vi "Heartbeat Checker.vi"(8 "Error In":errorcluster, 10 "Interval":i32=1000 format="%d ms", 11 "reference in":refnum<class "Network Mangement.lvclass">) -> ()   [LabVIEW 2024, in "Network Mangement.lvclass"]
uses:
  Network Mangement.lvclass
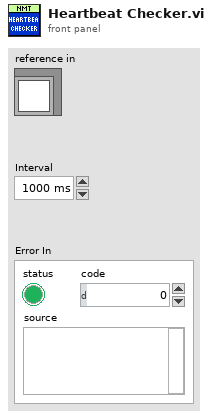
[diagram p1: front panel]
types:
  T1 = cluster{"Timeouted Heartbeat":cluster{"Node-ID":u8, "Heartbeat":cluster{"Period":u16, "Timeout":u16, "Last Beat":timestamp}}}
  T2 = typedef "Network Mangement.lvclass/ObjectAttributes.ctl" = cluster{"Nodes":map{u8, u8}, "Heartbeats":map{u8, cluster{"Period":u16, "Timeout":u16, "Last Beat":timestamp}}, "Events":cluster{"Stop Heartbeat Checker":refnum<user-event>, "Heartbeat Timeout":refnum<user-event>, "Heartbeat Checker Error":refnum<user-event>}, "Heartbeat Checker":refnum<vi>}
  T3 = map{u8, cluster{"Period":u16, "Timeout":u16, "Last Beat":timestamp}}
  T4 = cluster{"Period":u16, "Timeout":u16, "Last Beat":timestamp}
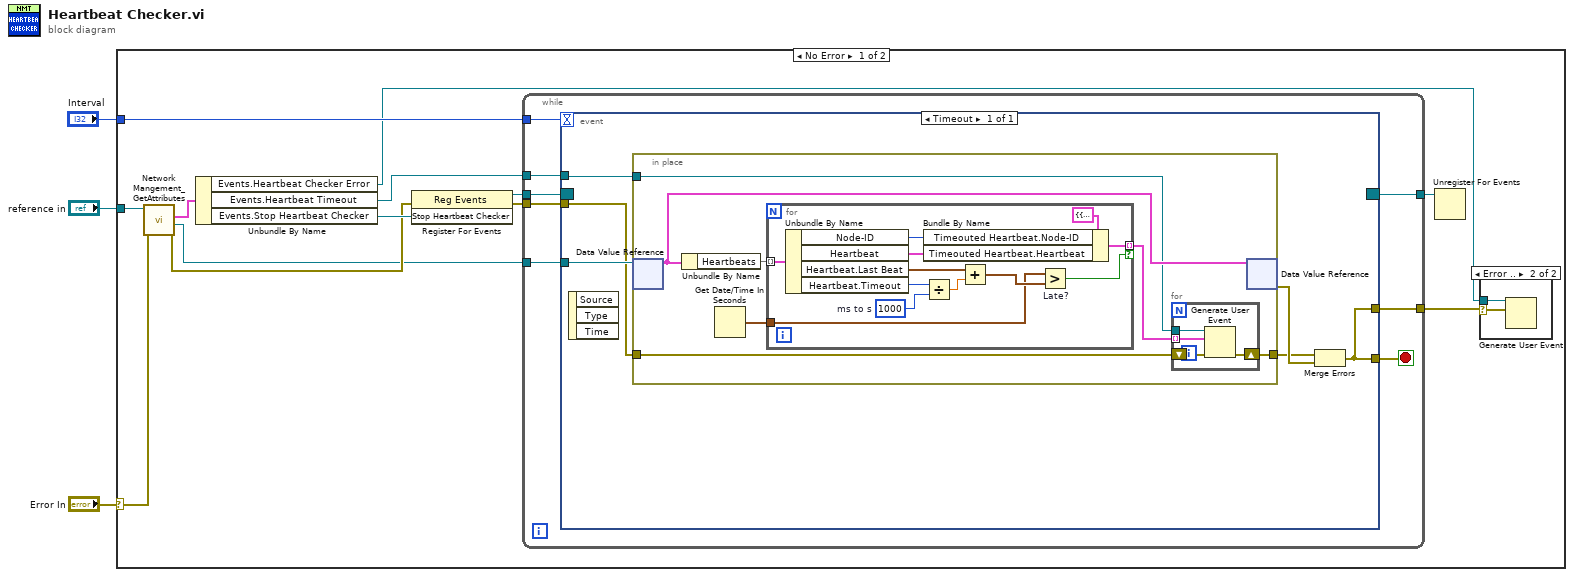
[diagram p0: block diagram]
diagram:
  n1 = case shown="No Error" "Error In" {
    selector: "Error In" -> [w16 _]
    tunnel: "reference in" -> [w14 _]
    tunnel: "Interval" -> [w10 _]
    frame No Error {
      n2 = call "Network Mangement_GetAttributes.vi"("Error In"=w16, "reference in"=w14) -> ("Error Out"=w12:errorcluster, "DataRef"=w8:refnum<data-value>, "Data"=w15:T2)  [unwired: 6 in, 1 out]
      n3 = Unbundle By Name(w15) -> ("Events.Heartbeat Checker Error"=w5:refnum<user-event>, "Events.Heartbeat Timeout"=w7:refnum<user-event>, "Events.Stop Heartbeat Checker"=w13:refnum<user-event>)
      n4 = register-events(error in=w12, w13) -> (reference out=w11:refnum<event-registration>, error out=w9:errorcluster)  [unwired: 1 in]
      n5 = while {
        tunnel: w11 -> [w24]
        tunnel: w10 -> [w23]
        tunnel: w9 -> [w22]
        tunnel: w8 -> [w21]
        tunnel: w7 -> [w19]
        tunnel: [w18] -> w4
        tunnel: [w17] -> w6
        stop <- w20 stop-if-true
        n6 = event shown="[0] Timeout" {
          selector: w24 -> [_]
          dyn-events: [_] -> w18
          timeout: w23 -> [_]
          tunnel: w22 -> [w27]
          tunnel: w21 -> [w30]
          tunnel: [w26] -> w20
          tunnel: w19 -> [w25]
          tunnel: [w26] -> w17
          event Timeout {
            n7 = event-data() -> ()  [unwired: 1 in, 3 out]
            n8 = in-place {
              in-place-border: [w32] -> w28
              in-place-border: w27 -> [w33]
              in-place-border: w25 -> [w34]
              n9 = in-place-dvr #1(w30) -> (w35:T2)  [unwired: 1 out]
              n10 = Unbundle By Name(w35) -> ("Heartbeats"=w37:T3)
              n11 = Get Date/Time In Seconds() -> (seconds since 1Jan1904=w36:timestamp)
              n12 = for {
                tunnel: w37 -> [w53] mode=indexing
                tunnel: w36 -> [w47]
                tunnel: [w43] -> w31 mode=indexing if=w42
                w51 = u16 1000  # ms to s
                n13 = Unbundle By Name(w53) -> ("Node-ID"=w45:u8, "Heartbeat"=w44:T4, "Heartbeat.Last Beat"=w49:timestamp, "Heartbeat.Timeout"=w52:u16)
                n14 = Bundle By Name(cluster=T1 {"Timeouted Heartbeat"={"Node-ID"=0, "Heartbeat"={"Period"=0, "Timeout"=0, "Last Beat"=timestamp(0 s since 1904-01-01)}}} ("event data"), "Timeouted Heartbeat.Node-ID"=w45, "Timeouted Heartbeat.Heartbeat"=w44) -> (w43:T1)
                n15 = Divide(x=w52, y=w51) -> (x/y=w50:dbl)
                n16 = Add(x=w49, y=w50) -> (x+y=w48:timestamp)
                n17 = Greater? "Late?"(x=w47, y=w48) -> (0:w42:bool)
              }
              n18 = for {
                tunnel: w34 -> [w41]
                tunnel: w31 -> [w38] mode=indexing
                shift-right: [w39] -> w32
                shift-left: w33 -> [w40]
                n19 = Generate User Event(user event=w41, event data cluster=w38, error in=w40) -> (error out=w39:errorcluster)  [unwired: 1 in, 1 out]
              }
              n20 = in-place-dvr #1(w35) -> (w29:errorcluster)  [unwired: 1 out]
            }
            n21 = Merge Errors(w28, w29) -> (w26:errorcluster)
          }
        }
      }
      n22 = Unregister For Events(event registration refnum=w4) -> ()  [unwired: 1 in, 1 out]
      n23 = case shown="Error .." w6 {
        selector: w6 -> [_ w54]
        tunnel: w5 -> [_ w55]
        frame No Error {
        }
        frame Error {
          n24 = Generate User Event(user event=w55, event data cluster=w54) -> ()  [unwired: 2 in, 2 out]
        }
      }
    }
    frame Error {
    }
  }
